vi "Channel Mng Performance Test.vi"() -> ()   [LabVIEW 2021]
uses:
  <vilib>/CIF Foundation/CIF Channels Core/CIFChannels/Typedef/Direction.ctl
  <vilib>/CIF Foundation/CIF Channels Core/CIFChannels/CIFChannels.lvclass/CIFChannels.ctl
  Channels/CIFChannelMng/CIFChannelMng.lvclass/CIFChannelMng.ctl
  <vilib>/CIF Foundation/NI Channels/SubVIs/Add Error.vi
  5cced918-02c8-46c6-a768-324ec32dc62f.vi/c28b0ead-42ad-4072-80a2-aca7f2bd7ce3.vi
  <vilib>/CIF Foundation/NI Channels/SubVIs/CIFServices Fill In Error Info Ex.vi
  <vilib>/CIF Foundation/NI Channels/SubVIs/Get dll Path.vi
  1c4ab14f-6bf4-49c1-a168-9d6ba27c2df9.vi/4bc1c15b-36ab-481f-b8dd-c64075ce723a.vi
  1c4ab14f-6bf4-49c1-a168-9d6ba27c2df9.vi/d83cb72b-7713-41fc-a3d1-682de79cf574.vi
  e632abc1-8e6e-452b-86d7-aafb18c83a30.vi/c28b0ead-42ad-4072-80a2-aca7f2bd7ce3.vi
  75b7e273-08cc-4638-a501-f0069bc9fa42.vi/c28b0ead-42ad-4072-80a2-aca7f2bd7ce3.vi
  75b7e273-08cc-4638-a501-f0069bc9fa42.vi/219d0231-d98b-4193-b5cc-84f90e3c9091.vi
  fb6d2954-3b48-4182-aeaa-f1d0ff0b1182.vi/c28b0ead-42ad-4072-80a2-aca7f2bd7ce3.vi
  fb6d2954-3b48-4182-aeaa-f1d0ff0b1182.vi/219d0231-d98b-4193-b5cc-84f90e3c9091.vi
  <vilib>/CIF Foundation/CIF Channels Core/CIFChannels/Accessors/Read Name.vi
  <vilib>/CIF Foundation/CIF Channels Core/CIFChannels/Accessors/Read Custom Config Data.vi
  <vilib>/CIF Foundation/CIF Channels Core/CIFChannels/Accessors/Read Type.vi
  <vilib>/CIF Foundation/CIF Channels Core/CIFChannels/Accessors/Read Pattern.vi
  <vilib>/CIF Foundation/CIF Channels Core/CIFChannels/Accessors/Read Direction.vi
  <vilib>/CIF Foundation/CIF Channels Core/CIFChannels/Accessors/Read Channel State.vi
  <vilib>/CIF Foundation/CIF Channels Core/ChannelCommon/Utilities/Add Error.vi
  Channels/CIFChannelMng/Utilities/Get Channel Index by Name.vi
  Channels/CIFChannelMng/Utilities/Remove Channel by Index.vi
  <vilib>/CIF Foundation/CIF Utilities/Errors/Append Error Location.vi
  <vilib>/CIF Foundation/CIF Channels Core/CIFChannels/Accessors/Write Channel State.vi
  <vilib>/CIF Foundation/CIF Channels Core/CIPC_Channels/Double/CIF_CIPC_Chn_Double.lvclass
  C:/Program Files/National Instruments/LabVIEW 2021/vi.lib/CIF Foundation/CIF Channels Core/CIFChannels/CIFChannels.lvclass
  <vilib>/CIF Foundation/CIF Channels Core/CIFChannels/CIFChannels.lvclass
  <vilib>/Platform/TimedLoop/XDataNode/wakeup.ctl
  <vilib>/Platform/TimedLoop/XDataNode/XDNodeRunTimeDep.lvlib
  <vilib>/Platform/TimedLoop/XDataNode/nitl_modes.ctl
  <vilib>/Platform/TimedLoop/XDataNode/timing_clust.ctl
  <vilib>/Platform/TimedLoop/XDataNode/XDataNode.xnode
  56cc47de-3fae-4a1e-b55c-fb66d6129849.vi
  a1e927e9-ff07-4866-b8c3-f0d77cb0f620.vi
  a6bb0a43-09af-4cb0-8e40-9eac7a17c1eb.vi
  09c8cd41-0623-4d79-8acb-fc72c701aad2.vi
  d3480e90-6007-42b0-867e-56b5d07abee3.vi
  <vilib>/CIF Foundation/NI Channels/NIChannels.lvlib
  <vilib>/CIF Foundation/CIF Channels Core/ChannelCommon/typedef/New FIFO Instance Response.ctl
  <vilib>/CIF Foundation/CIF Channels Core/ChannelCommon/ChannelCommon.lvlib
  Channels/CIFChannelMng/CIFChannelMng.lvclass
  C:/Program Files/National Instruments/LabVIEW 2021/vi.lib/CIF Foundation/CIF Channels Core/CIPC_Channels/CIF_CIPC_Chan/CIF_CIPC_Chn.lvclass
  C:/Program Files/National Instruments/LabVIEW 2021/vi.lib/CIF Foundation/CIF Channels Core/CIPC_Channels/Double/CIF_CIPC_Chn_Double.lvclass
panel:
  out "avg dbl channel":dbl
  out "max dbl channel":dbl
  in  "stop":bool
  out "avg raw channel":dbl
  out "max raw channel":dbl
  out "pass":bool
  out "error out":errorcluster
  # "This test should be run on RT.  It stresses the communications by constantly creating resource contraints with the low priority sender and the high priority loop. On Windows the priority of the loops cannot be set."
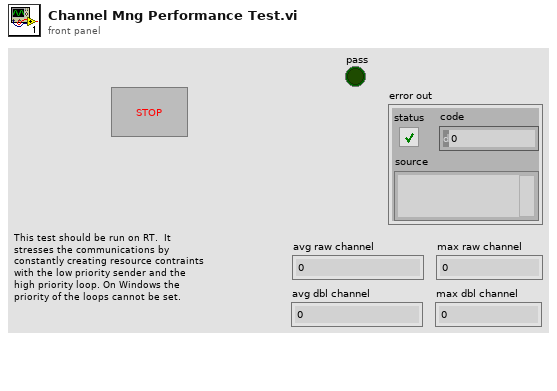
[diagram p1: front panel]
types:
  T1 = typedef "CIFChannels.lvclass/Direction.ctl" = enum16{"Publisher", "Subscriber"}
  T2 = typedef "XDNodeRunTimeDep.lvlib/timing_clust.ctl" = cluster{"Expected End [f-1]":u64, "Actual End [f-1]":u64, "Finished Late? [f-1]":bool, "Expected End [i-1]":u64, "Actual End [i-1]":u64, "Finished Late? [i-1]":bool, "Expected Start [i]":u64, "Actual Start [i]":u64, "Expected Start [f]":u64, "Actual Start [f]":u64, "Source Name":string, "Structure Name":string, "Period":i64, "Deadline":i64, "Offset":i64, "Start":i64, "Priority":i32, "Timeout":i32, "Mode":T3, "Wakeup Reason":T4, "Error":errorcluster, "Source Type":string, "Secondary Source Type":string, "Global End Time":u64, "Global Start Time":u64, "Frame Duration":u64, "Iteration Duration":u64, "Assigned CPU":i32, "I/O Scan Engine Mode":u32}
  T3 = typedef "XDNodeRunTimeDep.lvlib/nitl_modes.ctl" = enum32{"No Change", "Process missed periods, maintain original phase", "Discard missed periods, maintain original phase", "Process missed periods, ignore original phase", "Discard missed periods, ignore original phase"}
  T4 = typedef "XDNodeRunTimeDep.lvlib/wakeup.ctl" = enum32{"Normal", "Aborted", "Asynchronous wakeup", "Timing source error", "Timed loop error", "Timeout"}
  T5 = typedef "ChannelCommon.lvlib/New FIFO Instance Response.ctl" = cluster{"Publisher":string, "Custom Data":u8[]}
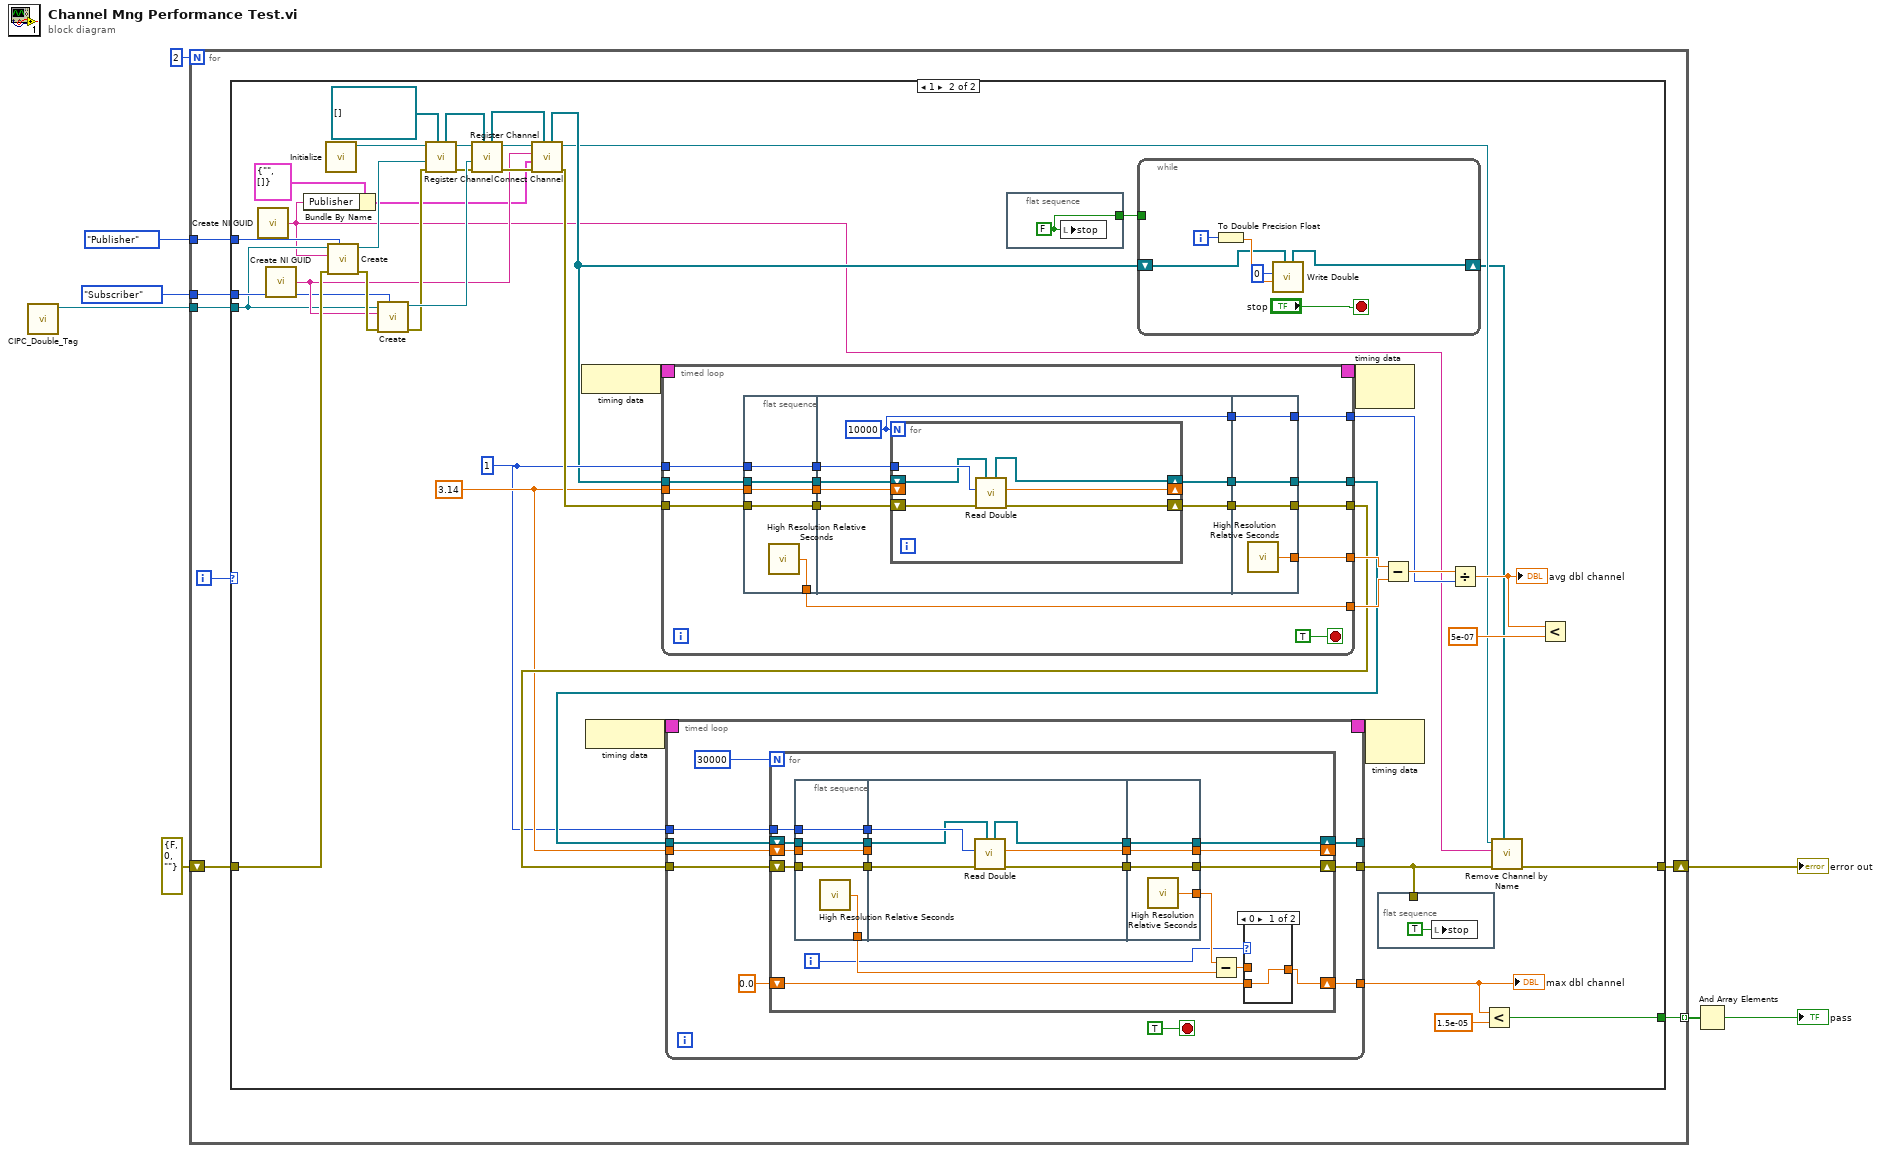
[diagram p0: block diagram]
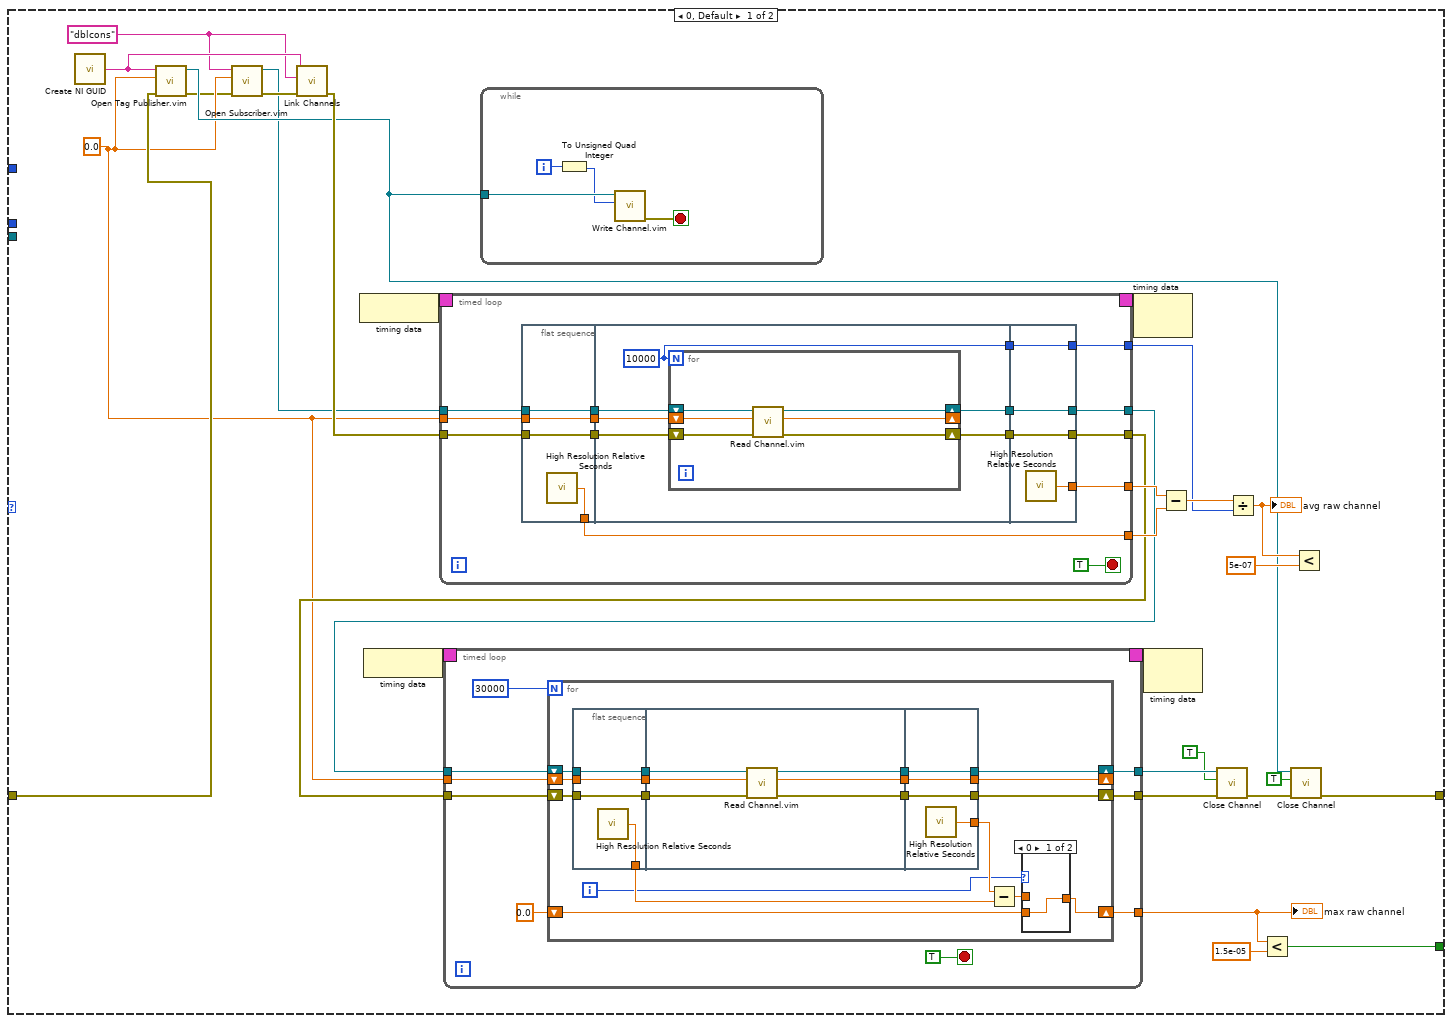
[diagram p2: hidden frame]
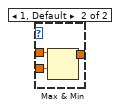
[diagram p3: hidden frame]
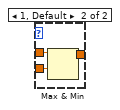
[diagram p4: hidden frame]
diagram:
  n1 = call <vilib>:"CIPC_Double_Tag.vi"() -> ("CIF_CIPC_Chn_Double.lvclass"=w4:refnum<class "CIF_CIPC_Chn_Double.lvclass">)  [unwired: 11 in]
  n2 = for {
    N: 2 -> [_]
    tunnel: [w15] -> w6 mode=indexing
    shift-right: [w14] -> w7
    shift-left: errorcluster {"status"=FALSE, "code"=0, "source"=""} ("error out") -> [w12]
    tunnel: Direction."Publisher" ("Direction") -> [w11]
    tunnel: Direction."Subscriber" ("Direction") -> [w10]
    tunnel: w4 -> [w9]
    i -> [w13]
    n3 = case shown="1" w13 {
      tunnel: [w31 w167] -> w15
      tunnel: [w24 w140] -> w14
      tunnel: w12 -> [w29 w158]
      tunnel: w11 -> [_ w154]
      tunnel: w10 -> [_ w153]
      tunnel: w9 -> [_ w152]
      frame 0, Default {
        w18 = "dblcons" ("Channel Name")
        w20 = 0.0
        n4 = call <vilib>:"Create NI GUID.vi"() -> ("NI GUID"=w22:string)
        n5 = call "Open Tag Publisher.vim"("error in"=w29, "Input Type"=w20, "Channel Name"=w22) -> ("error out"=w19:errorcluster, "CIF Channel"=w23:refnum<k21>)  [unwired: 7 in]
        n6 = call "Open Subscriber.vim"("error in"=w19, "Input Type"=w20, "Channel Name"=w18) -> ("error out"=w17:errorcluster, "CIF Channel"=w16:refnum<k21>)  [unwired: 7 in]
        n7 = call <vilib>:"Link Channels.vi"("error in"=w17, "Consumer Channel Name"=w18, "Producer Channel Name"=w22) -> ("error out"=w30:errorcluster)  [unwired: 8 in]
        n8 = node-c288() -> (w45:T2)
        n9 = node-c288() -> (w43:T2)
        n10 = timed-loop {
          timing: w45 -> [_]
          timing-out: [_] -> w44
          tunnel: w16 -> [w113]
          tunnel: w30 -> [w112]
          tunnel: [w108] -> w37
          tunnel: [w106] -> w36
          tunnel: [w104] -> w41
          tunnel: [w103] -> w40
          tunnel: [w102] -> w38
          tunnel: w20 -> [w100]
          stop <- TRUE stop-if-true
          n11 = flat-sequence {
            tunnel: w112 -> [w116]
            tunnel: w113 -> [w117]
            tunnel: [w117] -> w110
            tunnel: [w116] -> w109
            tunnel: [w115] -> w103
            tunnel: w100 -> [w114]
            tunnel: [w114] -> w99
            tunnel: w110 -> [w123]
            tunnel: w109 -> [w122]
            tunnel: [w121] -> w107
            tunnel: [w120] -> w105
            tunnel: [w119] -> w101
            tunnel: w99 -> [w118]
            tunnel: [w133] -> w108
            tunnel: w107 -> [w133]
            tunnel: [w132] -> w106
            tunnel: w105 -> [w132]
            tunnel: [w131] -> w104
            tunnel: [w130] -> w102
            tunnel: w101 -> [w130]
            frame #0 {
              n12 = call <vilib>:"High Resolution Relative Seconds.vi"() -> ("relative seconds"=w115:dbl)
            }
            frame #1 {
              w119 = 10000
              n13 = for {
                N: w119 -> [_]
                shift-right: [w126] -> w121
                shift-left: w123 -> [w129]
                shift-right: [w125] -> w120
                shift-left: w122 -> [w124]
                shift-right: [w127] -> _
                shift-left: w118 -> [w128]
                n14 = call "Read Channel.vim"("error in"=w124, "Data in"=w128, "CIF Channel in"=w129) -> ("error out"=w125:errorcluster, "Data out"=w127:dbl, "CIF Channel out"=w126:refnum<k21>)  [unwired: 5 in, 1 out]
              }
            }
            frame #2 {
              n15 = call <vilib>:"High Resolution Relative Seconds.vi"() -> ("relative seconds"=w131:dbl)
            }
          }
        }
        n16 = timed-loop {
          timing: w43 -> [_]
          timing-out: [_] -> w42
          tunnel: w37 -> [w58]
          tunnel: w36 -> [w57]
          tunnel: [w55] -> w27
          tunnel: [w54] -> w28
          tunnel: w20 -> [w53]
          tunnel: [w50] -> w33
          stop <- TRUE stop-if-true
          n17 = for {
            N: 30000 -> [_]
            shift-right: [w70] -> w55
            shift-left: w58 -> [w72]
            shift-right: [w69] -> w54
            shift-left: w57 -> [w71]
            shift-right: [w63] -> w50
            shift-left: 0.0 -> [w64]
            shift-right: [w62] -> _
            shift-left: w53 -> [w68]
            i -> [w60]
            n18 = flat-sequence {
              tunnel: w71 -> [w83]
              tunnel: w72 -> [w84]
              tunnel: [w84] -> w76
              tunnel: [w83] -> w75
              tunnel: [w82] -> w66
              tunnel: w68 -> [w81]
              tunnel: [w81] -> w74
              tunnel: w76 -> [w90]
              tunnel: w75 -> [w86]
              tunnel: [w89] -> w73
              tunnel: w74 -> [w88]
              tunnel: [w87] -> w61
              tunnel: [w85] -> w59
              tunnel: [w94] -> w70
              tunnel: w73 -> [w94]
              tunnel: [w93] -> w69
              tunnel: [w92] -> w67
              tunnel: [w91] -> w62
              tunnel: w61 -> [w91]
              tunnel: w59 -> [w93]
              frame #0 {
                n19 = call <vilib>:"High Resolution Relative Seconds.vi"() -> ("relative seconds"=w82:dbl)
              }
              frame #1 {
                n20 = call "Read Channel.vim"("error in"=w86, "Data in"=w88, "CIF Channel in"=w90) -> ("error out"=w85:errorcluster, "Data out"=w87:dbl, "CIF Channel out"=w89:refnum<k21>)  [unwired: 5 in, 1 out]
              }
              frame #2 {
                n21 = call <vilib>:"High Resolution Relative Seconds.vi"() -> ("relative seconds"=w92:dbl)
              }
            }
            n22 = Subtract(x=w67, y=w66) -> (x-y=w65:dbl)
            n23 = case shown="0" w60 {
              tunnel: w65 -> [_ w80]
              tunnel: w64 -> [w77 w79]
              tunnel: [w77 w78] -> w63
              frame 0 {
              }
              frame 1, Default {
                n24 = Max & Min(x=w80, y=w79) -> (max(x,y)=w78:dbl)  [unwired: 1 out]
              }
            }
          }
        }
        "max raw channel" <- w33
        n25 = while {
          tunnel: w23 -> [w48]
          i -> [w49]
          stop <- w46 stop-if-true
          n26 = To Unsigned Quad Integer(1:w49) -> (0:w47:u64)
          n27 = call "Write Channel.vim"("Data in"=w47, "CIF Channel in"=w48) -> ("error out"=w46:errorcluster)  [unwired: 6 in, 3 out]
        }
        n28 = node-c288(w44) -> ()  [unwired: 1 out]
        n29 = node-c288(w42) -> ()  [unwired: 1 out]
        n30 = Subtract(x=w41, y=w40) -> (x-y=w39:dbl)
        n31 = call <vilib>:"Close Channel.vi"("error in"=w28, "Force Destroy? (F)"=TRUE, "CIF Channel"=w27) -> ("error out"=w26:errorcluster)  [unwired: 8 in]
        n32 = Divide(x=w39, y=w38) -> (x/y=w35:dbl)
        "avg raw channel" <- w35
        n33 = Less?(x=w33, y=1.5e-05) -> (x < y?=w31:bool)
        n34 = call <vilib>:"Close Channel.vi"("error in"=w26, "Force Destroy? (F)"=TRUE, "CIF Channel"=w23) -> ("error out"=w24:errorcluster)  [unwired: 8 in]
        n35 = Less?(x=w35, y=5e-07) -> ()  [unwired: 1 out]
      }
      frame 1 {
        w151 = 1 ("Channel Index")
        w156 = 3.14 ("Default Value")
        n36 = call <vilib>:"Create NI GUID.vi"() -> ("NI GUID"=w143:string)
        n37 = call <vilib>:"Create NI GUID.vi"() -> ("NI GUID"=w155:string)
        n38 = Bundle By Name(cluster=T5 {"Publisher"="", "Custom Data"=[]} ("Connection"), "Publisher"=w143) -> (w142:T5)
        n39 = call "Initialize.vi"() -> ("CIFChannelMng out"=w150:refnum<class "CIFChannelMng.lvclass">)  [unwired: 10 in, 1 out]
        n40 = call-dynamic "Create.vi"("Direction"=w154, "error in (no error)"=w158, "Name"=w143, "CIFTag in"=w152) -> ("error out"=w162:errorcluster, "CIFTag out"=w161:refnum<class "CIF_CIPC_Chn_Double.lvclass">)  [unwired: 6 in]
        n41 = call-dynamic "Create.vi"("Direction"=w153, "error in (no error)"=w162, "Name"=w155, "CIFTag in"=w152) -> ("error out"=w163:errorcluster, "CIFTag out"=w166:refnum<class "CIF_CIPC_Chn_Double.lvclass">)  [unwired: 6 in]
        n42 = call "Register Channel.vi"("Channel Array in"=refnum<class "CIFChannels.lvclass">[] [], "error in (no error)"=w163, "Channel"=w161, "CIFChannelMng in"=w150) -> ("error out"=w160:errorcluster, "CIFChannelMng out"=w159:refnum<class "CIFChannelMng.lvclass">, "Channel Array out"=w148:refnum<class "CIFChannels.lvclass">[])  [unwired: 4 in, 1 out]
        n43 = call "Register Channel.vi"("Channel Array in"=w148, "error in (no error)"=w160, "Channel"=w166, "CIFChannelMng in"=w159) -> ("error out"=w165:errorcluster, "CIFChannelMng out"=w164:refnum<class "CIFChannelMng.lvclass">, "Channel Array out"=w147:refnum<class "CIFChannels.lvclass">[])  [unwired: 4 in, 1 out]
        n44 = call "Connect Channel.vi"("Channel Array in"=w147, "error in (no error)"=w165, "Connection"=w142, "Subscriber Name"=w155, "CIFChannelMng in"=w164) -> ("error out"=w157:errorcluster, "CIFChannelMng out"=w145:refnum<class "CIFChannelMng.lvclass">, "Channel Array out"=w146:refnum<class "CIFChannels.lvclass">[])  [unwired: 3 in, 1 out]
        n45 = node-c288() -> (w181:T2)
        n46 = node-c288() -> (w179:T2)
        n47 = timed-loop {
          timing: w181 -> [_]
          timing-out: [_] -> w180
          tunnel: w146 -> [w259]
          tunnel: w157 -> [w258]
          tunnel: [w254] -> w173
          tunnel: [w252] -> w172
          tunnel: [w250] -> w177
          tunnel: [w249] -> w176
          tunnel: [w248] -> w174
          tunnel: w156 -> [w246]
          tunnel: w151 -> [w244]
          stop <- TRUE stop-if-true
          n48 = flat-sequence {
            tunnel: w258 -> [w263]
            tunnel: w259 -> [w264]
            tunnel: [w264] -> w256
            tunnel: [w263] -> w255
            tunnel: [w262] -> w249
            tunnel: w246 -> [w261]
            tunnel: [w261] -> w245
            tunnel: w244 -> [w260]
            tunnel: [w260] -> w243
            tunnel: w256 -> [w271]
            tunnel: w255 -> [w270]
            tunnel: [w269] -> w253
            tunnel: [w268] -> w251
            tunnel: [w267] -> w247
            tunnel: w245 -> [w266]
            tunnel: w243 -> [w265]
            tunnel: [w281] -> w254
            tunnel: w253 -> [w281]
            tunnel: [w280] -> w252
            tunnel: w251 -> [w280]
            tunnel: [w279] -> w250
            tunnel: [w278] -> w248
            tunnel: w247 -> [w278]
            frame #0 {
              n49 = call <vilib>:"High Resolution Relative Seconds.vi"() -> ("relative seconds"=w262:dbl)
            }
            frame #1 {
              w267 = 10000
              n50 = for {
                N: w267 -> [_]
                shift-right: [w272] -> w269
                shift-left: w271 -> [w273]
                shift-right: [w277] -> w268
                shift-left: w270 -> [w276]
                shift-right: [w275] -> _
                shift-left: w266 -> [_]
                tunnel: w265 -> [w274]
                n51 = call "Read Double.vi"("Channel Array in"=w273, "error in (no error)"=w276, "Channel Index"=w274) -> ("error out"=w277:errorcluster, "Data"=w275:dbl, "Channel Array out"=w272:refnum<class "CIFChannels.lvclass">[])  [unwired: 5 in, 1 out]
              }
            }
            frame #2 {
              n52 = call <vilib>:"High Resolution Relative Seconds.vi"() -> ("relative seconds"=w279:dbl)
            }
          }
        }
        n53 = timed-loop {
          timing: w179 -> [_]
          timing-out: [_] -> w178
          tunnel: w173 -> [w199]
          tunnel: w172 -> [w198]
          tunnel: [w196] -> _
          tunnel: [w195] -> w139
          tunnel: w156 -> [w194]
          tunnel: [w191] -> w169
          tunnel: w151 -> [w190]
          stop <- TRUE stop-if-true
          n54 = for {
            N: 30000 -> [_]
            shift-right: [w213] -> w196
            shift-left: w199 -> [w215]
            shift-right: [w212] -> w195
            shift-left: w198 -> [w214]
            shift-right: [w206] -> w191
            shift-left: 0.0 -> [w207]
            shift-right: [w205] -> _
            shift-left: w194 -> [w211]
            tunnel: w190 -> [w201]
            i -> [w203]
            n55 = flat-sequence {
              tunnel: w214 -> [w227]
              tunnel: w215 -> [w228]
              tunnel: [w228] -> w219
              tunnel: [w227] -> w218
              tunnel: [w226] -> w209
              tunnel: w211 -> [w225]
              tunnel: [w225] -> w217
              tunnel: w201 -> [w224]
              tunnel: [w224] -> w200
              tunnel: w219 -> [w230]
              tunnel: w218 -> [w234]
              tunnel: [w229] -> w216
              tunnel: w217 -> [_]
              tunnel: [w232] -> w204
              tunnel: [w233] -> w202
              tunnel: w200 -> [w231]
              tunnel: [w238] -> w213
              tunnel: w216 -> [w238]
              tunnel: [w237] -> w212
              tunnel: [w236] -> w210
              tunnel: [w235] -> w205
              tunnel: w204 -> [w235]
              tunnel: w202 -> [w237]
              frame #0 {
                n56 = call <vilib>:"High Resolution Relative Seconds.vi"() -> ("relative seconds"=w226:dbl)
              }
              frame #1 {
                n57 = call "Read Double.vi"("Channel Array in"=w230, "error in (no error)"=w234, "Channel Index"=w231) -> ("error out"=w233:errorcluster, "Data"=w232:dbl, "Channel Array out"=w229:refnum<class "CIFChannels.lvclass">[])  [unwired: 5 in, 1 out]
              }
              frame #2 {
                n58 = call <vilib>:"High Resolution Relative Seconds.vi"() -> ("relative seconds"=w236:dbl)
              }
            }
            n59 = Subtract(x=w210, y=w209) -> (x-y=w208:dbl)
            n60 = case shown="0" w203 {
              tunnel: w208 -> [_ w223]
              tunnel: w207 -> [w220 w222]
              tunnel: [w220 w221] -> w206
              frame 0 {
              }
              frame 1, Default {
                n61 = Max & Min(x=w223, y=w222) -> (max(x,y)=w221:dbl)  [unwired: 1 out]
              }
            }
          }
        }
        "max dbl channel" <- w169
        n62 = flat-sequence {
          tunnel: [w183] -> w141
          frame #0 {
            w183 = FALSE ("stop")
            n63 = local write "stop"(w183) -> ()
          }
        }
        n64 = while {
          shift-right: [w185] -> w138
          shift-left: w146 -> [w186]
          tunnel: w141 -> [_]
          i -> [w189]
          stop <- "stop" stop-if-true
          n65 = To Double Precision Float(number=w189) -> (double precision float=w188:dbl)
          n66 = call "Write Double.vi"("Channel Array in"=w186, "Data"=w188, "Channel Index"=0) -> ("Channel Array out"=w185:refnum<class "CIFChannels.lvclass">[])  [unwired: 6 in, 2 out]
        }
        n67 = node-c288(w180) -> ()  [unwired: 1 out]
        n68 = node-c288(w178) -> ()  [unwired: 1 out]
        n69 = flat-sequence {
          tunnel: w139 -> [_]
          frame #0 {
            n70 = local write "stop"(TRUE ("stop")) -> ()
          }
        }
        n71 = Subtract(x=w177, y=w176) -> (x-y=w175:dbl)
        n72 = Divide(x=w175, y=w174) -> (x/y=w171:dbl)
        "avg dbl channel" <- w171
        n73 = Less?(x=w169, y=1.5e-05) -> (x < y?=w167:bool)
        n74 = call "Remove Channel by Name.vi"("Channel Array in"=w138, "error in (no error)"=w139, "Channel Name"=w143, "CIFChannelMng in"=w145) -> ("error out"=w140:errorcluster)  [unwired: 4 in, 3 out]
        n75 = Less?(x=w171, y=5e-07) -> ()  [unwired: 1 out]
      }
    }
  }
  "error out" <- w7
  n76 = And Array Elements(Boolean array=w6) -> (logical AND=→"pass":bool)
